vi "Form_additionall_str.vi"(1 "Array":string[](array[string])) -> (0 "String":string)   [LabVIEW 2020]
panel:
  out "Numeric":i32
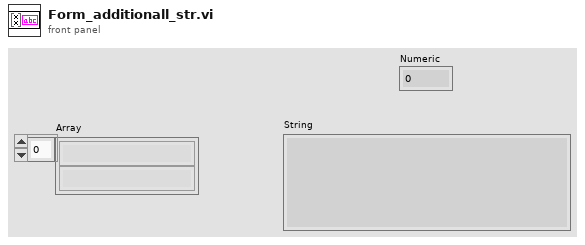
[diagram p1: front panel]
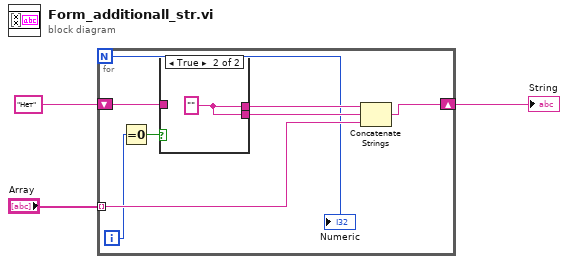
[diagram p0: block diagram]
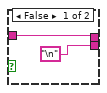
[diagram p2: hidden frame]
diagram:
  n1 = for {
    N -> [w4]
    tunnel: "Array" -> [w10] mode=indexing
    shift-right: [w9] -> w1
    shift-left: "Нет" -> [w7]
    i -> [w5]
    n2 = Equal To 0?(x=w5) -> (x = 0?=w6:bool)
    n3 = case shown="True" w6 {
      tunnel: ["\n" w14] -> w11
      tunnel: [w13 w14] -> w8
      tunnel: w7 -> [w13 _]
      frame False {
      }
      frame True {
        w14 = "" ("f")
      }
    }
    n4 = Concatenate Strings(w8, w11, w10) -> (w9:string)
    "Numeric" <- w4
  }
  "String" <- w1
